vi "LogSort_Stack.vi"(0 "Function":enum16{"Init", "Push", "Pop", "Size"}(ring), 1 "Indices":cluster{"First":i32, "Last":i32}, 3 "Size":i32=1024) -> (15 "Indices":cluster{"First":i32, "Last":i32}, 17 "Size":i32)   [LabVIEW 2011, in "i3-oauth-logicalstringarraysort.lvlib"]
uses:
  i3-oauth-logicalstringarraysort.lvlib
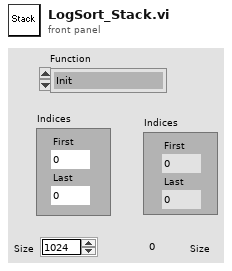
[diagram p1: front panel]
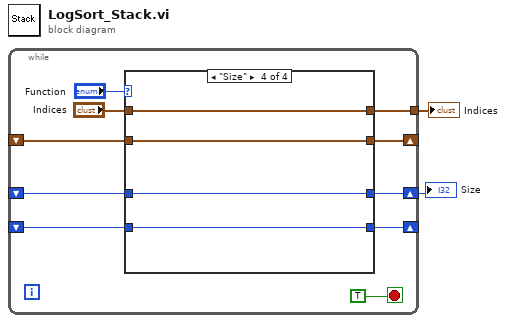
[diagram p0: block diagram]
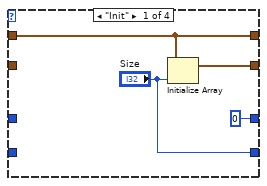
[diagram p2: hidden frame]
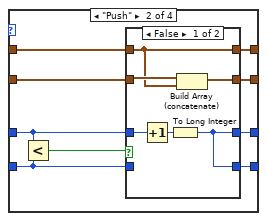
[diagram p3: hidden frame]
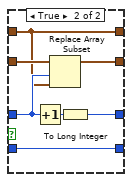
[diagram p4: hidden frame]
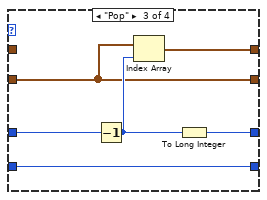
[diagram p5: hidden frame]
diagram:
  n1 = while {
    shift-left: _ -> [w4]
    shift-right: [w5] -> _
    shift-left: _ -> [w7]
    shift-right: [w6] -> w1
    tunnel: [w9] -> w2
    shift-left: _ -> [w10]
    shift-right: [w11] -> _
    stop <- TRUE stop-if-true
    n2 = case shown="\"Size\"" "Function" {
      tunnel: [w16 w23 w40 w46] -> w11
      tunnel: w10 -> [_ w24 w40 w46]
      tunnel: "Indices" -> [w15 w18 _ w48]
      tunnel: [w15 w17 w44 w48] -> w9
      tunnel: w7 -> [_ w22 w43 w47]
      tunnel: [0 w25 w42 w47] -> w6
      tunnel: ["Size" w19 w39 w45] -> w5
      tunnel: w4 -> [_ w20 w39 w45]
      frame "Init" {
        n3 = Initialize Array(w15, "Size") -> (w16:cluster{"First":i32, "Last":i32}[])
      }
      frame "Push" {
        n4 = Less?(x=w22, y=w20) -> (x < y?=w21:bool)
        n5 = case shown="False" w21 {
          tunnel: w22 -> [w31 w38]
          tunnel: w18 -> [w26 w32]
          tunnel: [w28 w36] -> w23
          tunnel: w24 -> [w27 w35]
          tunnel: [w29 w34] -> w25
          tunnel: w20 -> [_ w33]
          tunnel: [w29 w33] -> w19
          tunnel: [w26 w32] -> w17
          frame False {
            n6 = Increment(x=w31) -> (x+1=w30:i32)
            n7 = To Long Integer(number=w30) -> (32bit integer=w29:i32)
            n8 = Build Array (concatenate)(w27, w26) -> (w28:cluster{"First":i32, "Last":i32}[])
          }
          frame True {
            n9 = Increment(x=w38) -> (x+1=w37:i32)
            n10 = Replace Array Subset(array=w35, new element=w32, index=w38) -> (w36:cluster{"First":i32, "Last":i32}[])
            n11 = To Long Integer(number=w37) -> (32bit integer=w34:i32)
          }
        }
      }
      frame "Pop" {
        n12 = Decrement(x=w43) -> (x-1=w41:i32)
        n13 = Index Array(array=w40, index=w41) -> (element=w44:cluster{"First":i32, "Last":i32})
        n14 = To Long Integer(number=w41) -> (32bit integer=w42:i32)
      }
      frame "Size" {
      }
    }
  }
  "Indices" <- w2
  "Size" <- w1
